vi "Write Status Source.vi"(8 "error in (no error)":errorcluster, 10 "Status Source":T1, 11 "VisaComms in":refnum<class "VisaComms.lvclass">) -> (0 "error out":errorcluster, 3 "VisaComms out":refnum<class "VisaComms.lvclass">)   [LabVIEW 2024, in "CTI.lvlib" / "VisaComms.lvclass"]
uses:
  VisaComms.lvclass
  Status Source.ctl
  VisaComms.lvclass/VisaComms.ctl
  Clean Visa Errors.vi
  CTI.lvlib
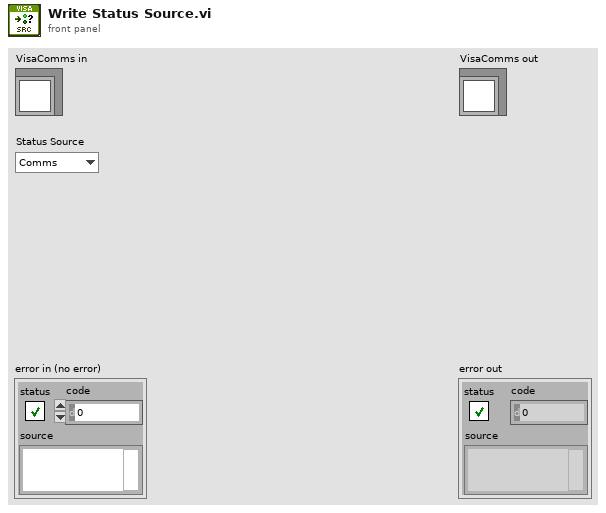
[diagram p1: front panel]
types:
  T1 = typedef "CTI.lvlib/Status Source.ctl" = enum16{"Comms", "User"}
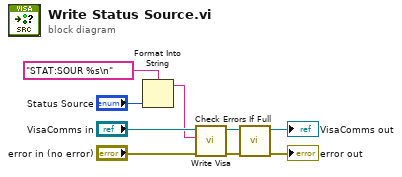
[diagram p0: block diagram]
diagram:
  n1 = Format Into String(format string="STAT:SOUR %s\n", "Status Source") -> (resulting string=w4:string)  [unwired: 2 in, 1 out]
  n2 = call "Write Visa.vi"("error in (no error)"="error in (no error)", "write buffer"=w4, "VisaComms in"="VisaComms in") -> ("error out"=w2:errorcluster, "VisaComms out"=w8:refnum<class "VisaComms.lvclass">)  [unwired: 6 in, 1 out]
  n3 = call "Check Errors If Full.vi"("error in (no error)"=w2, "VisaComms in"=w8) -> ("error out"=→"error out":errorcluster, "VisaComms out"=→"VisaComms out":refnum<class "VisaComms.lvclass">)  [unwired: 8 in]
